vi "Display spectroscopy.vi"(8 "ALL harmonics phase 3":dbl[][](graph)=array1356x8[10848 elements], 11 "ALL harmonics mag":dbl[][](graph)=array1356x8[10848 elements]) -> ()   [LabVIEW 2021]
uses:
  <vilib>/Analysis/NI_AALBase.lvlib
panel:
  out "Baseline":cdb[](array[numeric])
  out "ALL harmonics \nmag BC":dbl[][](graph)
  in  "Scale.Range:Maximum 16":dbl=3e-05 format="%#_6p"
  in  "Scale.Range:Maximum 15":dbl=3e-05 format="%#_6p"
  in  "Scale.Range:Maximum 14":dbl=3e-05 format="%#_6p"
  in  "Scale.Range:Maximum 13":dbl=3e-05 format="%#_6p"
  in  "Scale.Range:Maximum 12":dbl=3e-05 format="%#_6p"
  in  "Scale.Range:Maximum 11":dbl=3e-05 format="%#_6p"
  in  "Scale.Range:Maximum 10":dbl=3e-05 format="%#_6p"
  in  "Scale.Range:Maximum 9":dbl=3e-05 format="%#_6p"
  in  "Scale.Range:Maximum 8":dbl=1e-05 format="%#_6p"
  in  "Scale.Range:Maximum 7":dbl=1e-05 format="%#_6p"
  in  "Scale.Range:Maximum 6":dbl=1e-05 format="%#_6p"
  in  "Scale.Range:Maximum 5":dbl=1e-05 format="%#_6p"
  in  "Scale.Range:Maximum 4":dbl=1e-05 format="%#_6p"
  in  "Scale.Range:Maximum 3":dbl=1e-05 format="%#_6p"
  in  "Scale.Range:Maximum 2":dbl=1e-05 format="%#_6p"
  in  "Scale.Range:Maximum":dbl=1e-05 format="%#_6p"
  in  "N":dbl=10.0
  out "9f0 3":dbl=4.0104772933755055e-07 format="%#_2p"
  out "8f0 3":dbl=3.538211619276352e-07 format="%#_2p"
  out "7f0 3":dbl=2.725951794271453e-07 format="%#_2p"
  out "6f0 3":dbl=3.090424281975066e-07 format="%#_2p"
  out "5f0 3":dbl=2.299086519401267e-07 format="%#_2p"
  out "4f0 3":dbl=2.2412086738435062e-07 format="%#_2p"
  out "3f0 3":dbl=3.174604432569019e-07 format="%#_2p"
  out "2f0 3":dbl=2.0718928376888083e-07 format="%#_2p"
  out "9f0_TankStd":dbl(slide)=4.0104772933755055e-07 scale=1e-07..3e-05 scale format="%#_2p"
  out "8f0_TankStd":dbl(slide)=3.538211619276352e-07 scale=1e-07..3e-05 scale format="%#_2p"
  out "7f0_TankStd":dbl(slide)=2.725951794271453e-07 scale=1e-07..3e-05 scale format="%#_2p"
  out "6f0_TankStd":dbl(slide)=3.090424281975066e-07 scale=1e-07..3e-05 scale format="%#_2p"
  out "5f0_TankStd":dbl(slide)=2.299086519401267e-07 scale=1e-07..3e-05 scale format="%#_2p"
  out "3f0_TankStd":dbl(slide)=3.174604432569019e-07 scale=0.0..3e-05 scale format="%#_2p"
  out "4f0_TankStd":dbl(slide)=2.2412086738435062e-07 scale=1e-07..3e-05 scale format="%#_2p"
  out "2f0_TankStd":dbl(slide)=2.0718928376888083e-07 scale=1e-07..3e-05 scale format="%#_2p"
  out "9f0":dbl=5.709143822073392e-07 format="%#_2p"
  out "8f0":dbl=7.215800050274871e-07 format="%#_2p"
  out "7f0":dbl=6.575500482955872e-07 format="%#_2p"
  out "6f0":dbl=5.762406086855072e-07 format="%#_2p"
  out "5f0":dbl=5.419265654611816e-07 format="%#_2p"
  out "4f0":dbl=5.063464549948812e-07 format="%#_2p"
  out "3f0":dbl=8.836385712157283e-07 format="%#_2p"
  out "2f0":dbl=4.553165861737233e-07 format="%#_2p"
  out "9f0_Tank":dbl(slide)=5.709143822073392e-07 scale=1e-07..1e-05 scale format="%#_2p"
  out "8f0_Tank":dbl(slide)=7.215800050274871e-07 scale=1e-07..1e-05 scale format="%#_2p"
  out "7f0_Tank":dbl(slide)=6.575500482955872e-07 scale=1e-07..1e-05 scale format="%#_2p"
  out "6f0_Tank":dbl(slide)=5.762406086855072e-07 scale=1e-07..1e-05 scale format="%#_2p"
  out "5f0_Tank":dbl(slide)=5.419265654611816e-07 scale=1e-07..1e-05 scale format="%#_2p"
  out "4f0_Tank":dbl(slide)=5.063464549948812e-07 scale=1e-07..1e-05 scale format="%#_2p"
  out "3f0_Tank":dbl(slide)=8.836385712157283e-07 scale=1e-07..1e-05 scale format="%#_2p"
  out "2f0_Tank":dbl(slide)=4.553165861737233e-07 scale=1e-07..1e-05 scale format="%#_2p"
  # "Mean\nLast N Pts"
  # "Std\nLast N Pts"
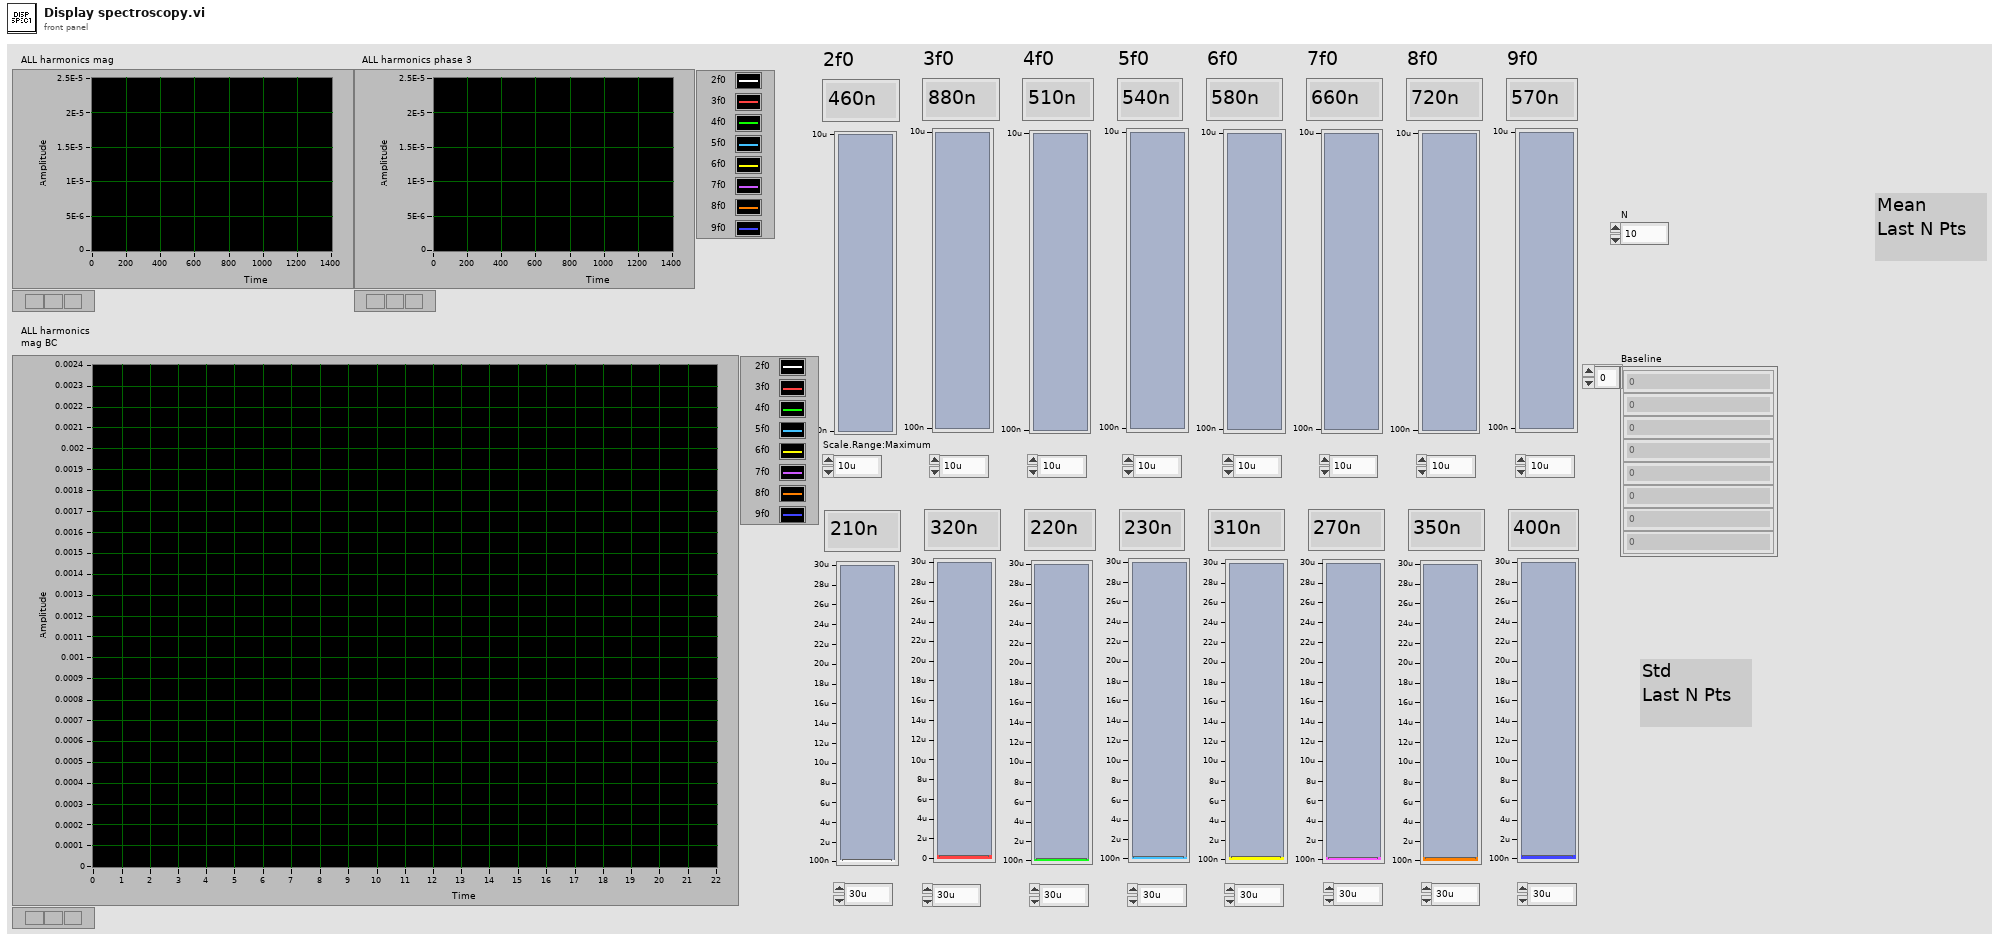
[diagram p1: front panel]
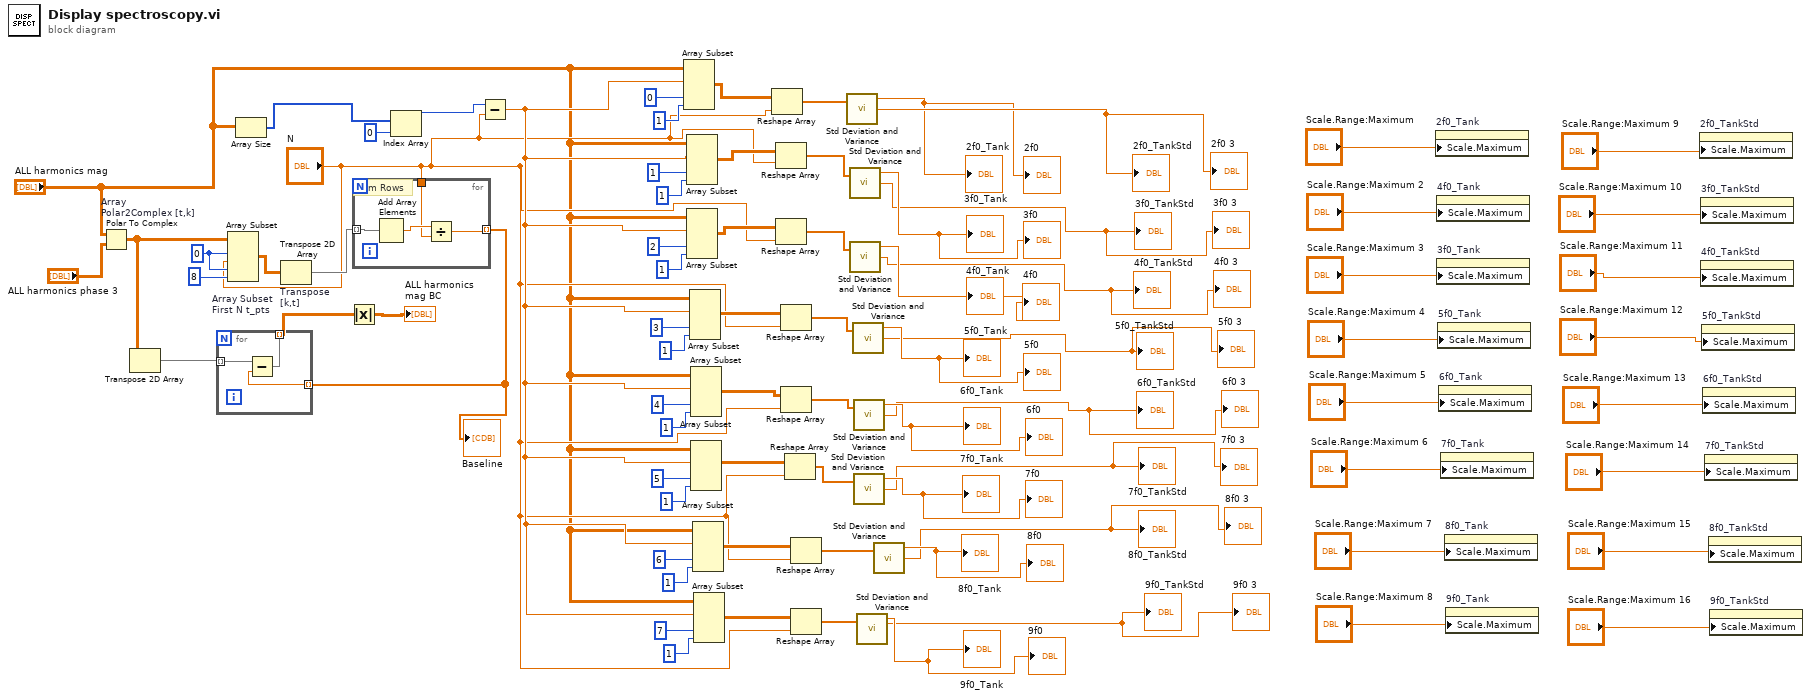
[diagram p0: block diagram]
diagram:
  w9 = 0
  n1 = Polar To Complex "Array \nPolar2Complex [t,k]"(1:"ALL harmonics phase 3", 2:"ALL harmonics mag") -> (0:w4:cdb[][])
  n2 = Transpose 2D Array(2D array=w4) -> (transposed array=w3:cdb[][])
  n3 = Array Subset "Array Subset\nFirst N t_pts"(array=w4, index (row)=w9, length (row)="N", index (col)=w9, length (col)=8) -> (w7:cdb[][])
  n4 = Array Size(array="ALL harmonics mag") -> (size(s)=w80:i32[])
  n5 = Transpose 2D Array "Transpose\n[k,t]"(2D array=w7) -> (transposed array=w10:cdb[][])
  n6 = for {
    tunnel: w10 -> [w84] mode=indexing
    tunnel: [w82] -> w5 mode=indexing
    tunnel: "N" -> [w81]
    # "Sum Rows"
    n7 = Add Array Elements(numeric array=w84) -> (sum=w83:cdb)
    n8 = Divide(x=w83, y=w81) -> (x/y=w82:cdb)
  }
  "Baseline" <- w5
  n9 = for {
    tunnel: w3 -> [w87] mode=indexing
    tunnel: w5 -> [w86] mode=indexing
    tunnel: [w85] -> w2 mode=indexing
    n10 = Subtract(x=w87, y=w86) -> (x-y=w85:cdb[])
  }
  n11 = Absolute Value(x=w2) -> (abs(x)=→"ALL harmonics \nmag BC":dbl[][])
  n12 = Index Array(array=w80, index=0) -> (element=w75:i32)
  n13 = Subtract(x=w75, y="N") -> (x-y=w46:dbl)
  n14 = Array Subset(array="ALL harmonics mag", index (row)=w46, index (col)=0, length (col)=1) -> (w43:dbl[][])  [unwired: 1 in]
  n15 = Array Subset(array="ALL harmonics mag", index (row)=w46, index (col)=1, length (col)=1) -> (w41:dbl[][])  [unwired: 1 in]
  n16 = Array Subset(array="ALL harmonics mag", index (row)=w46, index (col)=2, length (col)=1) -> (w40:dbl[][])  [unwired: 1 in]
  n17 = Array Subset(array="ALL harmonics mag", index (row)=w46, index (col)=3, length (col)=1) -> (w37:dbl[][])  [unwired: 1 in]
  n18 = Array Subset(array="ALL harmonics mag", index (row)=w46, index (col)=4, length (col)=1) -> (w36:dbl[][])  [unwired: 1 in]
  n19 = Array Subset(array="ALL harmonics mag", index (row)=w46, index (col)=5, length (col)=1) -> (w33:dbl[][])  [unwired: 1 in]
  n20 = Array Subset(array="ALL harmonics mag", index (row)=w46, index (col)=6, length (col)=1) -> (w32:dbl[][])  [unwired: 1 in]
  n21 = Array Subset(array="ALL harmonics mag", index (row)=w46, index (col)=7, length (col)=1) -> (w29:dbl[][])  [unwired: 1 in]
  n22 = Reshape Array(w43, "N") -> (w44:dbl[])
  n23 = Reshape Array(w41, "N") -> (w42:dbl[])
  n24 = Reshape Array(w40, "N") -> (w39:dbl[])
  n25 = Reshape Array(w37, "N") -> (w38:dbl[])
  n26 = Reshape Array(w36, "N") -> (w35:dbl[])
  n27 = Reshape Array(w33, "N") -> (w34:dbl[])
  n28 = Reshape Array(w32, "N") -> (w31:dbl[])
  n29 = Reshape Array(w29, "N") -> (w30:dbl[])
  n30 = call <vilib>:"Std Deviation and Variance.vi"("X"=w44) -> ("mean"=→"2f0_Tank" →"2f0":dbl, "standard deviation"=→"2f0_TankStd" →"2f0 3":dbl)  [unwired: 1 in, 1 out]
  n31 = call <vilib>:"Std Deviation and Variance.vi"("X"=w42) -> ("mean"=→"3f0_Tank" →"3f0":dbl, "standard deviation"=→"3f0_TankStd" →"3f0 3":dbl)  [unwired: 1 in, 1 out]
  n32 = call <vilib>:"Std Deviation and Variance.vi"("X"=w39) -> ("mean"=→"4f0_Tank" →"4f0":dbl, "standard deviation"=→"4f0_TankStd" →"4f0 3":dbl)  [unwired: 1 in, 1 out]
  n33 = call <vilib>:"Std Deviation and Variance.vi"("X"=w38) -> ("mean"=→"5f0_Tank" →"5f0":dbl, "standard deviation"=→"5f0_TankStd" →"5f0 3":dbl)  [unwired: 1 in, 1 out]
  n34 = call <vilib>:"Std Deviation and Variance.vi"("X"=w35) -> ("mean"=→"6f0_Tank" →"6f0":dbl, "standard deviation"=→"6f0_TankStd" →"6f0 3":dbl)  [unwired: 1 in, 1 out]
  n35 = call <vilib>:"Std Deviation and Variance.vi"("X"=w34) -> ("mean"=→"7f0_Tank" →"7f0":dbl, "standard deviation"=→"7f0_TankStd" →"7f0 3":dbl)  [unwired: 1 in, 1 out]
  n36 = call <vilib>:"Std Deviation and Variance.vi"("X"=w30) -> ("mean"=→"9f0_Tank" →"9f0":dbl, "standard deviation"=→"9f0_TankStd" →"9f0 3":dbl)  [unwired: 1 in, 1 out]
  n37 = call <vilib>:"Std Deviation and Variance.vi"("X"=w31) -> ("mean"=→"8f0_Tank" →"8f0":dbl, "standard deviation"=→"8f0_TankStd" →"8f0 3":dbl)  [unwired: 1 in, 1 out]
  n38 = property on="2f0_Tank" class="Slide (strict)"("Scale.Maximum"="Scale.Range:Maximum") -> ()  [unwired: 2 in, 2 out]
  n39 = property on="4f0_Tank" class="Slide (strict)"("Scale.Maximum"="Scale.Range:Maximum 2") -> ()  [unwired: 2 in, 2 out]
  n40 = property on="3f0_Tank" class="Slide (strict)"("Scale.Maximum"="Scale.Range:Maximum 3") -> ()  [unwired: 2 in, 2 out]
  n41 = property on="5f0_Tank" class="Slide (strict)"("Scale.Maximum"="Scale.Range:Maximum 4") -> ()  [unwired: 2 in, 2 out]
  n42 = property on="6f0_Tank" class="Slide (strict)"("Scale.Maximum"="Scale.Range:Maximum 5") -> ()  [unwired: 2 in, 2 out]
  n43 = property on="7f0_Tank" class="Slide (strict)"("Scale.Maximum"="Scale.Range:Maximum 6") -> ()  [unwired: 2 in, 2 out]
  n44 = property on="8f0_Tank" class="Slide (strict)"("Scale.Maximum"="Scale.Range:Maximum 7") -> ()  [unwired: 2 in, 2 out]
  n45 = property on="9f0_Tank" class="Slide (strict)"("Scale.Maximum"="Scale.Range:Maximum 8") -> ()  [unwired: 2 in, 2 out]
  n46 = property on="2f0_TankStd" class="Slide (strict)"("Scale.Maximum"="Scale.Range:Maximum 9") -> ()  [unwired: 2 in, 2 out]
  n47 = property on="3f0_TankStd" class="Slide (strict)"("Scale.Maximum"="Scale.Range:Maximum 10") -> ()  [unwired: 2 in, 2 out]
  n48 = property on="4f0_TankStd" class="Slide (strict)"("Scale.Maximum"="Scale.Range:Maximum 11") -> ()  [unwired: 2 in, 2 out]
  n49 = property on="5f0_TankStd" class="Slide (strict)"("Scale.Maximum"="Scale.Range:Maximum 12") -> ()  [unwired: 2 in, 2 out]
  n50 = property on="6f0_TankStd" class="Slide (strict)"("Scale.Maximum"="Scale.Range:Maximum 13") -> ()  [unwired: 2 in, 2 out]
  n51 = property on="7f0_TankStd" class="Slide (strict)"("Scale.Maximum"="Scale.Range:Maximum 14") -> ()  [unwired: 2 in, 2 out]
  n52 = property on="8f0_TankStd" class="Slide (strict)"("Scale.Maximum"="Scale.Range:Maximum 15") -> ()  [unwired: 2 in, 2 out]
  n53 = property on="9f0_TankStd" class="Slide (strict)"("Scale.Maximum"="Scale.Range:Maximum 16") -> ()  [unwired: 2 in, 2 out]
